vi "Obtain Semaphores.vi"(8 "error in (no error)":errorcluster, 10 "VI refs in":refnum<vi>[](array[refnum]), 11 "Slave Test Runner In":refnum<class "Slave Test Runner.lvclass">) -> (0 "error out":errorcluster, 2 "VI Refs out":refnum<vi>[](array[refnum]), 3 "Slave Test Runner Out":refnum<class "Slave Test Runner.lvclass">)   [LabVIEW 2020, in "Slave Test Runner.lvclass"]
uses:
  Slave Test Runner.lvclass
  Slave Test Runner.lvclass/Slave Test Runner.ctl
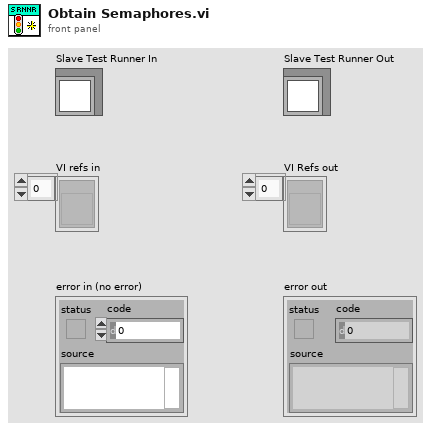
[diagram p1: front panel]
types:
  T1 = typedef "Semaphore RefNum" = refnum<k1>
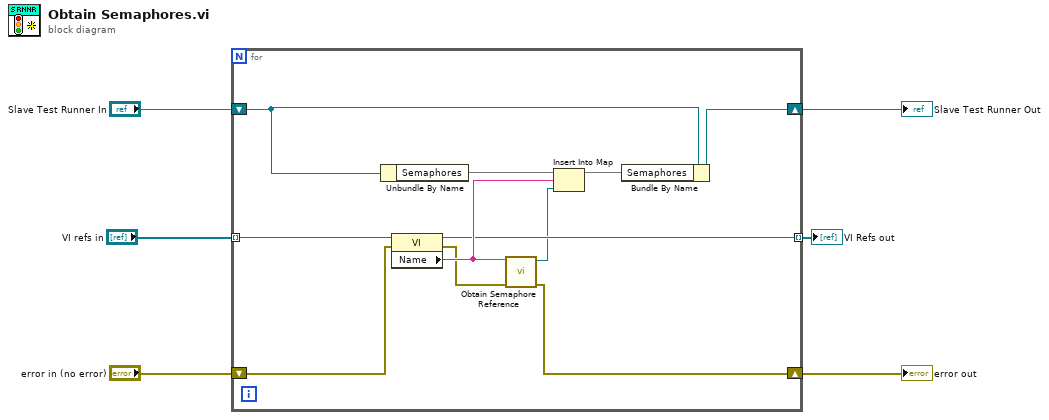
[diagram p0: block diagram]
diagram:
  n1 = for {
    shift-right: [w15] -> w5
    shift-left: "Slave Test Runner In" -> [w16]
    shift-right: [w10] -> w3
    shift-left: "error in (no error)" -> [w13]
    tunnel: "VI refs in" -> [w9] mode=indexing
    tunnel: [w8] -> w1 mode=indexing
    n2 = Unbundle By Name(w16) -> ("Semaphores"=w17:map{string, T1})
    n3 = property on="Property Node" class="VI"(reference=w9, error in=w13) -> (reference out=w8:refnum<vi>, error out=w11:errorcluster, "Name"=w12:string)
    n4 = call <vilib>:"Obtain Semaphore Reference.vi"("error in (no error)"=w11, "name (unnamed)"=w12) -> ("error out"=w10:errorcluster, "semaphore"=w7:T1)  [unwired: 3 in, 1 out]
    n5 = Insert Into Map(map in=w17, key=w12, value=w7) -> (map out=w14:map{string, T1})  [unwired: 2 out]
    n6 = Bundle By Name(cluster=w16, "Semaphores"=w14) -> (w15:refnum<class "Slave Test Runner.lvclass">)
  }
  "error out" <- w3
  "Slave Test Runner Out" <- w5
  "VI Refs out" <- w1
